vi "Packet Decode.vi"(8 "error in (no error)":errorcluster, 10 "Data":u8[](array[numeric]), 11 "Packet in":refnum<class "Packet.lvclass">) -> (0 "error out":errorcluster, 3 "Packet out":refnum<class "Packet.lvclass">)   [LabVIEW 2019, in "Packet.lvclass"]
uses:
  Packet.lvclass
  packet type STYP.ctl
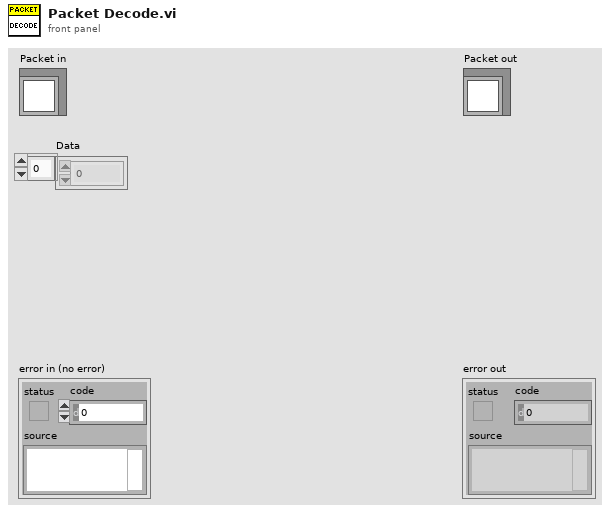
[diagram p1: front panel]
types:
  T1 = typedef "Packet.lvclass/packet type STYP.ctl" = enum16{"Connect", "Disconnect", "Direction", "Score", "Map"}
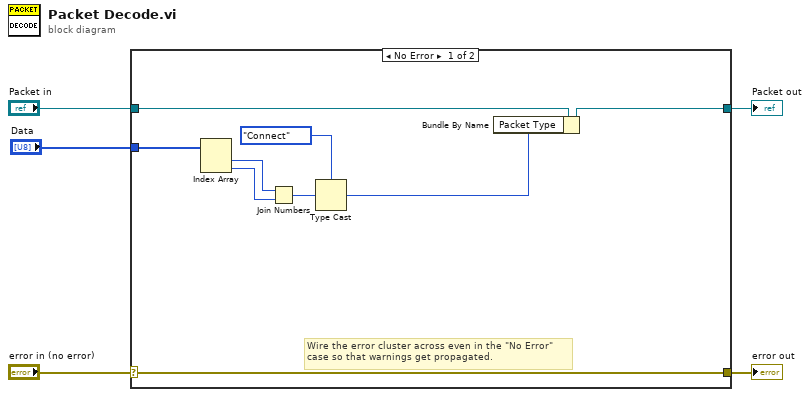
[diagram p0: block diagram]
diagram:
  n1 = case shown="No Error" "error in (no error)" {
    selector: "error in (no error)" -> [w13 w16]
    tunnel: [w13 w16] -> w4
    tunnel: [w7 w15] -> w2
    tunnel: "Packet in" -> [w14 w15]
    tunnel: "Data" -> [w12 _]
    frame No Error {
      # "Wire the error cluster across even in the \"No Error\"\ncase so that warnings get propagated."
      n2 = Index Array(array=w12) -> (element #1=w11:u8, element #2=w10:u8)  [unwired: 2 in]
      n3 = Join Numbers(hi=w11, lo=w10) -> ((hi.lo)=w9:u16)
      n4 = Type Cast(type=packet_type_STYP."Connect" ("Enum"), x=w9) -> (*(type *) &x=w6:T1)
      n5 = Bundle By Name(cluster=w14, "Packet Type"=w6) -> (w7:refnum<class "Packet.lvclass">)
    }
    frame Error {
    }
  }
  "error out" <- w4
  "Packet out" <- w2
